vi "PMX_GetDeviceStatus.vi"(8 "Error in":errorcluster, 11 "Device":refnum<k24>) -> (0 "Error out":errorcluster, 2 "DeviceStatus":i32, 3 "Device":refnum<k24>)   [LabVIEW 2016]
doc: "Returns the current status of the device"
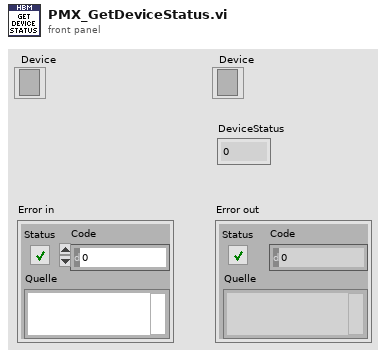
[diagram p1: front panel]
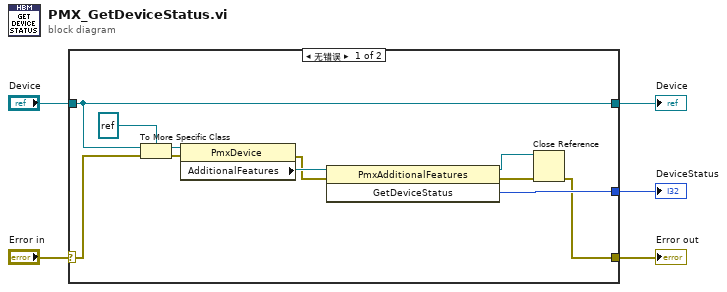
[diagram p0: block diagram]
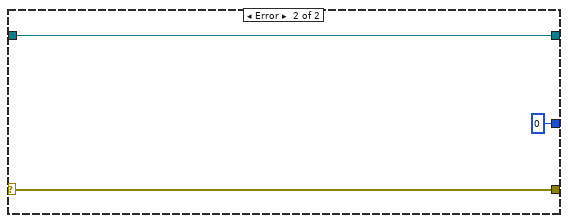
[diagram p2: hidden frame]
diagram:
  n1 = case shown="无错误" "Error in" {
    selector: "Error in" -> [w10 w19]
    tunnel: [w7 w19] -> w3
    tunnel: "Device" -> [w11 w18]
    tunnel: [w12 0 ("GetDeviceStatus")] -> w1
    tunnel: [w11 w18] -> w4
    frame No Error {
      n2 = To More Specific Class(target class=refnum<k24> refnum ("Zielklasse"), reference=w11, error in=w10) -> (specific class reference=w16:refnum<k24>, error out=w13:errorcluster)
      n3 = property on="Eigenschaftsknoten" class="PmxDevice"(reference=w16, error in=w13) -> (error out=w14:errorcluster, "AdditionalFeatures"=w15:refnum<k24>)  [unwired: 1 out]
      n4 = invoke on="Methodenknoten" class="PmxAdditionalFeatures" method="GetDeviceStatus"(reference=w15, error in=w14) -> (reference out=w6:refnum<k24>, error out=w8:errorcluster, "GetDeviceStatus"=w12:i32)  [unwired: 1 in]
      n5 = Close Reference(reference=w6, error in (no error)=w8) -> (error out=w7:errorcluster)
    }
    frame Error {
    }
  }
  "Device" <- w4
  "Error out" <- w3
  "DeviceStatus" <- w1
